vi "Test U8 Change FIFO Size.vi"() -> ()   [LabVIEW 2021]
uses:
  CIFChannels/Typedef/Direction.ctl
  ChannelCommon/typedef/FIFO Config.ctl
  ChannelCommon/typedef/TimeStamps.ctl
  CIF_CIPC_Fifo_U8.lvclass
  D:/dev/Packages/CIF_Channels_Core/src/CIPC_Channels/CIF_CIPC_Chan/CIF_CIPC_Chn.lvclass
  D:/dev/Packages/CIF_Channels_Core/src/CIFChannels/CIFChannels.lvclass
  ChannelCommon/typedef/New FIFO Instance Configuration.ctl
  CIFChannels/CIFChannels.lvclass/CIFChannels.ctl
  CIFChannels/Accessors/Read Publisher Name.vi
  <vilib>/CIF Foundation/CIF Utilities/DataTypes/Flatten Unflatten/Flatten U64.vi
  CIF_CIPC_Chan/CIF_CIPC_Chn.lvclass
  ChannelCommon/ChannelCommon.lvlib
  CIFChannels/CIFChannels.lvclass
panel:
  out "status":string
  out "pass":bool
  out "error out":errorcluster
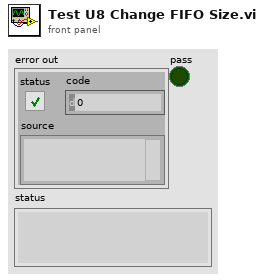
[diagram p1: front panel]
types:
  T1 = typedef "CIFChannels.lvclass/Direction.ctl" = enum16{"Publisher", "Subscriber"}
  T2 = typedef "ChannelCommon.lvlib/New FIFO Instance Configuration.ctl" = cluster{"Backpressure":bool, "Bytes/Message Override":u32, "Messages/FIFO Override":u32, "Custom Data":u8[]}
  T3 = typedef "ChannelCommon.lvlib/TimeStamps.ctl" = cluster{"ClockID":u8, "T0":i64, "T_Out":i64}
  T4 = typedef "ChannelCommon.lvlib/FIFO Config.ctl" = cluster{"Max Bytes/Msg":u64, "Max Msg/FIFO":u64, "Flags":u64}
  T5 = typedef "ChannelCommon.lvlib/New FIFO Instance Response.ctl" = cluster{"Publisher":string, "Custom Data":u8[]}
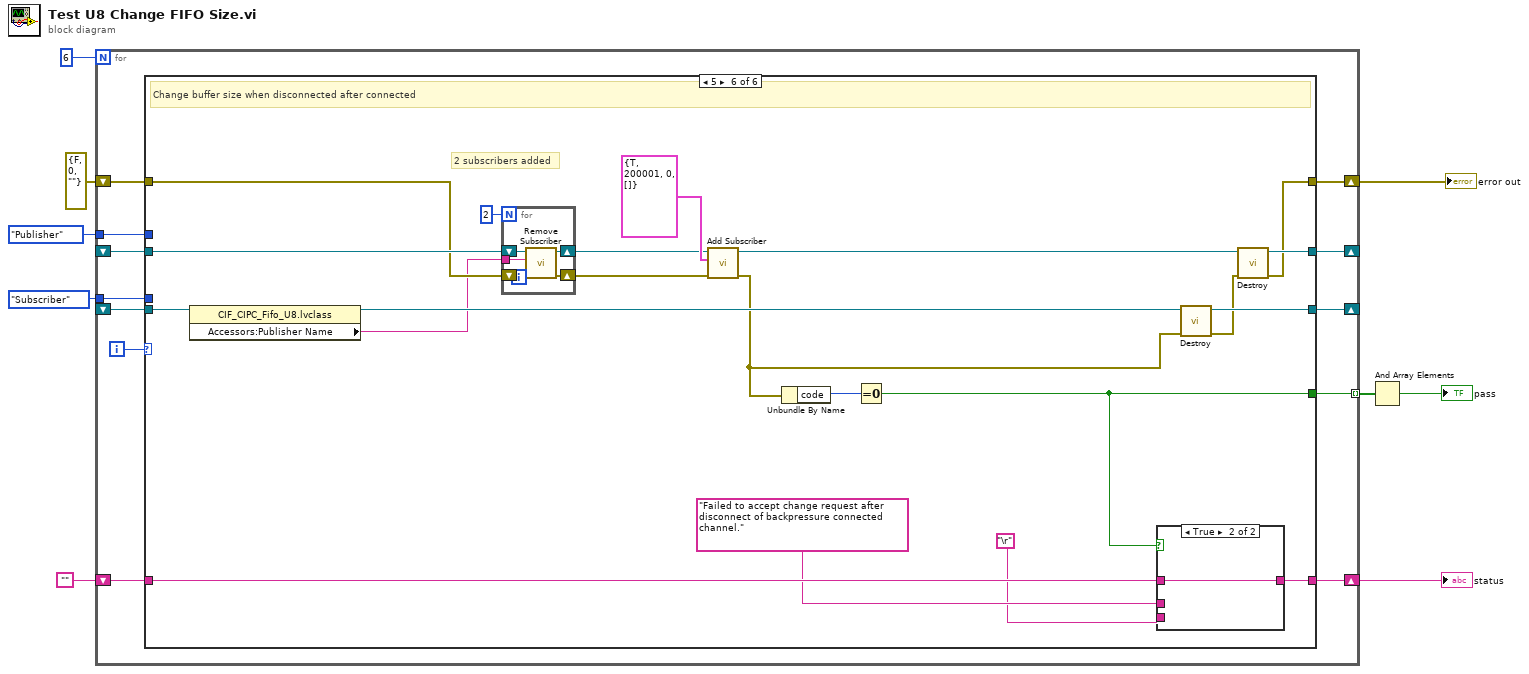
[diagram p0: block diagram]
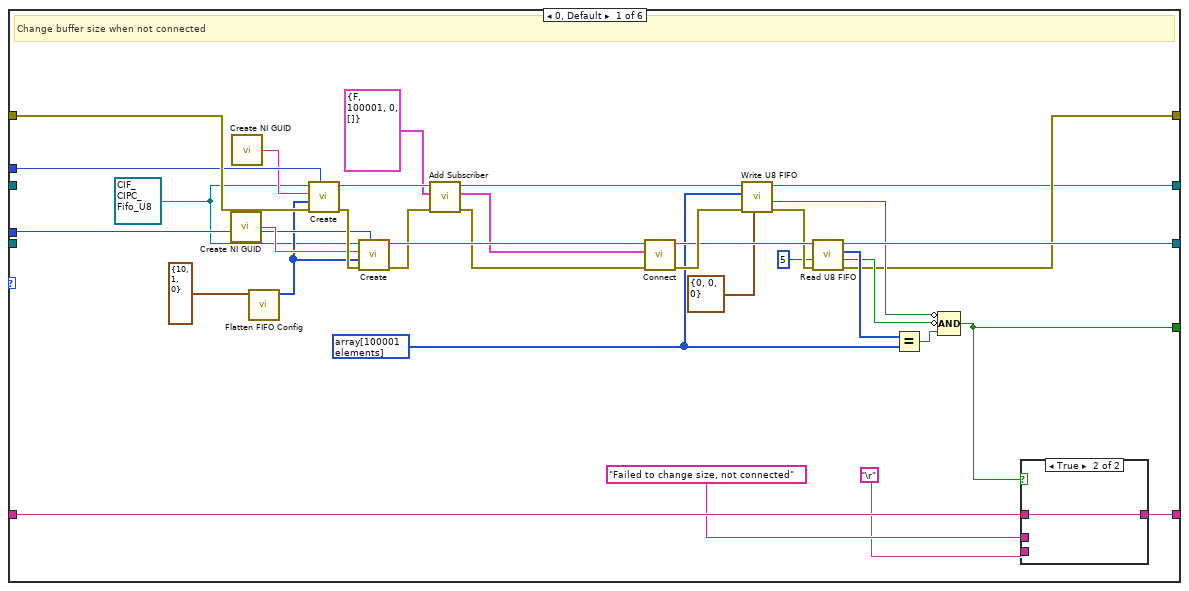
[diagram p2: hidden frame]
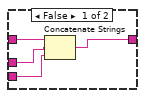
[diagram p3: hidden frame]
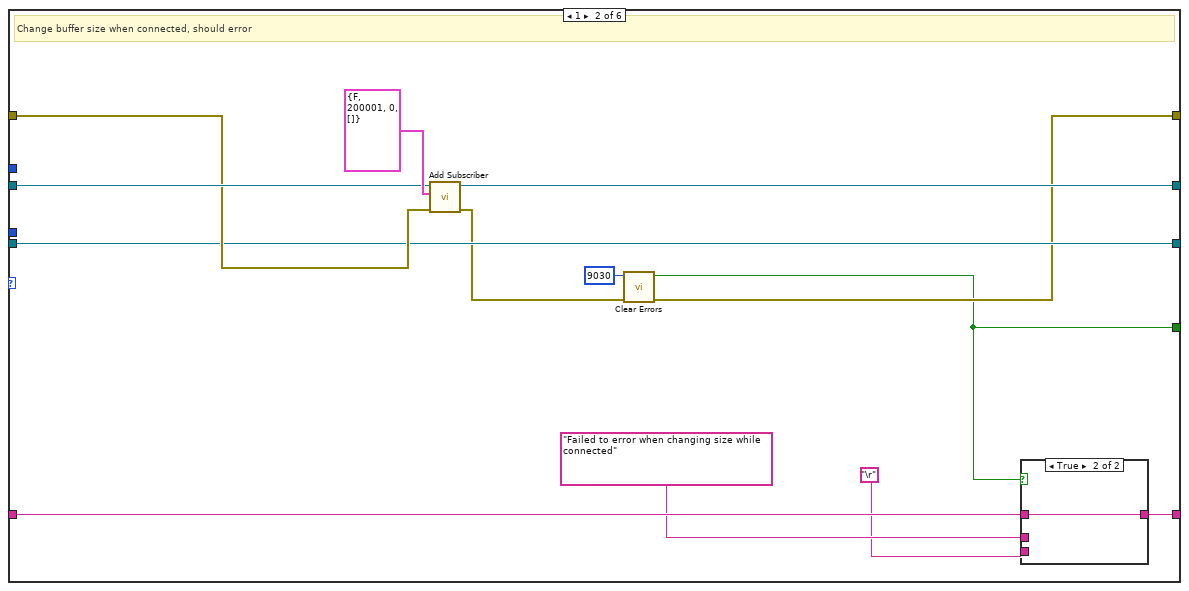
[diagram p4: hidden frame]
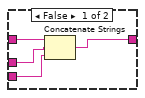
[diagram p5: hidden frame]
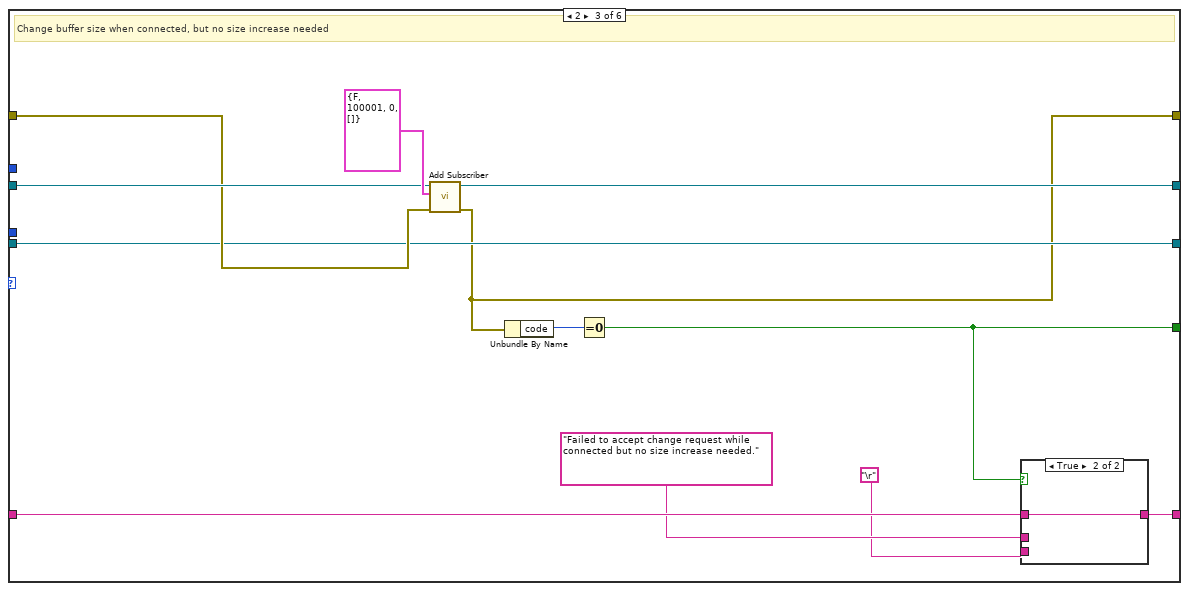
[diagram p6: hidden frame]
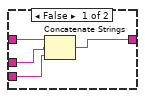
[diagram p7: hidden frame]
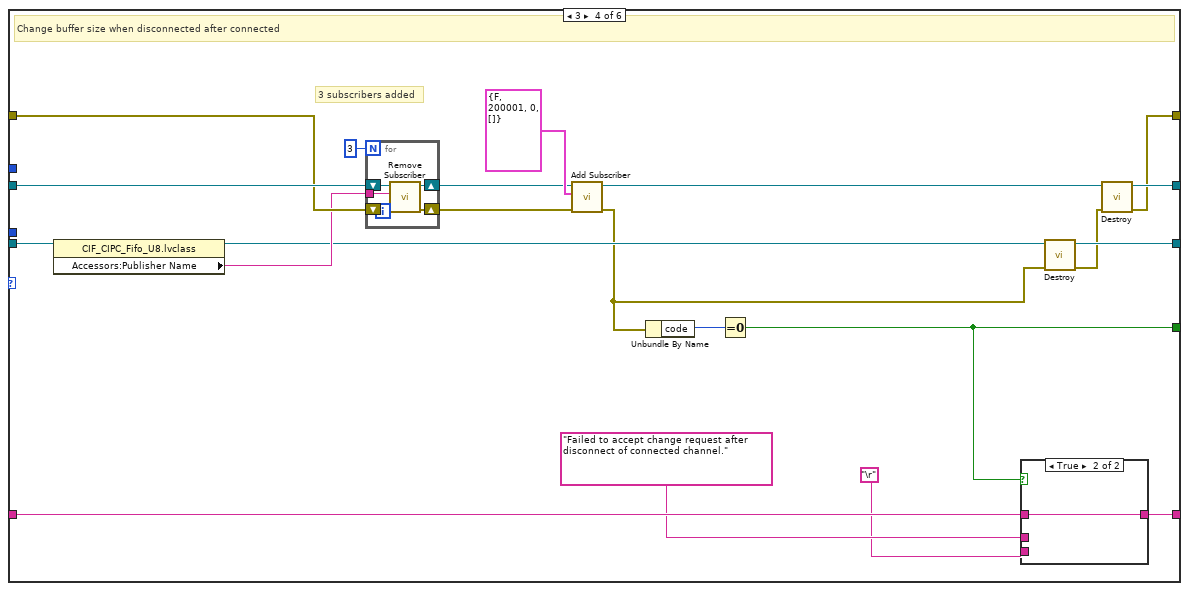
[diagram p8: hidden frame]
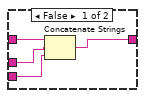
[diagram p9: hidden frame]
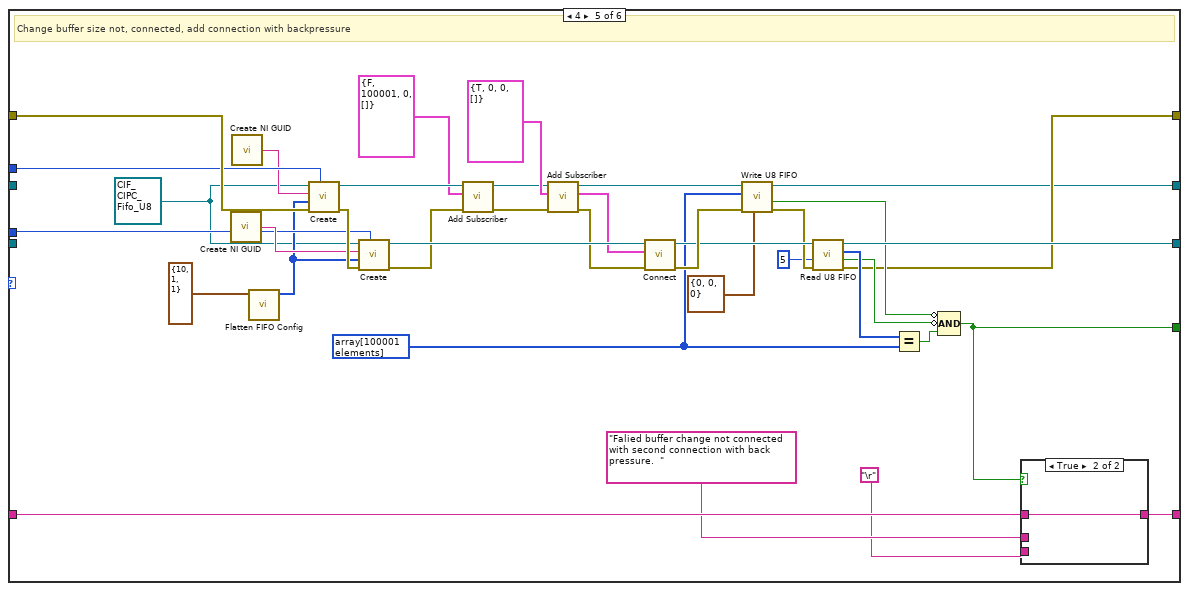
[diagram p10: hidden frame]
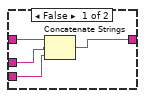
[diagram p11: hidden frame]
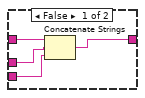
[diagram p12: hidden frame]
diagram:
  n1 = for {
    N: 6 -> [_]
    tunnel: [w21] -> w9 mode=indexing
    shift-right: [w19] -> w1
    shift-left: errorcluster {"status"=FALSE, "code"=0, "source"=""} ("error out") -> [w20]
    shift-right: [w16] -> w5
    shift-left: "" -> [w17]
    tunnel: Direction."Subscriber" ("Direction") -> [w15]
    tunnel: Direction."Publisher" ("Direction") -> [w14]
    shift-right: [w13] -> _
    shift-left: _ -> [w11]
    shift-right: [w12] -> _
    shift-left: _ -> [w10]
    i -> [w18]
    n2 = case shown="5" w18 {
      tunnel: [w50 w61 w79 w110 w158 w183] -> w21
      tunnel: w20 -> [w48 w67 w84 w106 w156 w179]
      tunnel: [w29 w63 w81 w96 w137 w170] -> w19
      tunnel: w17 -> [w55 w73 w90 w116 w163 w189]
      tunnel: [w54 w72 w89 w115 w162 w188] -> w16
      tunnel: w15 -> [w46 _ _ _ w154 _]
      tunnel: w14 -> [w45 _ _ _ w153 _]
      tunnel: [w39 w66 w83 w100 w147 w174] -> w13
      tunnel: [w28 w65 w82 w99 w136 w173] -> w12
      tunnel: w10 -> [_ w68 w85 w109 _ w182]
      tunnel: w11 -> [_ w66 w83 w105 _ w178]
      frame 0, Default {
        w33 = refnum<class "CIF_CIPC_Fifo_U8.lvclass"> refnum ("CIF_CIPC_Fifo_U8.lvclass")
        w30 = u8[] array[100001 elements] ("U8 Data")
        # "Change buffer size when not connected"
        n3 = call <vilib>:"Create NI GUID.vi"() -> ("NI GUID"=w47:string)
        n4 = call <vilib>:"Create NI GUID.vi"() -> ("NI GUID"=w43:string)
        n5 = call "Flatten FIFO Config.vi"("FIFO Config in"=T4 {"Max Bytes/Msg"=10, "Max Msg/FIFO"=1, "Flags"=0}) -> ("Flattened FIFO Config"=w34:u8[])  [unwired: 10 in]
        n6 = call-dynamic "Create.vi"("Direction"=w45, "error in (no error)"=w48, "Custom Config Data"=w34, "Name"=w43, "CIFFIFO in"=w33) -> ("error out"=w49:errorcluster, "CIFFIFO out"=w27:refnum<class "CIF_CIPC_Fifo_U8.lvclass">)  [unwired: 5 in]
        n7 = call-dynamic "Create.vi"("Direction"=w46, "error in (no error)"=w49, "Custom Config Data"=w34, "Name"=w47, "CIFFIFO in"=w33) -> ("error out"=w23:errorcluster, "CIFFIFO out"=w42:refnum<class "CIF_CIPC_Fifo_U8.lvclass">)  [unwired: 5 in]
        n8 = call-dynamic "Add Subscriber.vi"("error in (no error)"=w23, "New FIFO Instance Config"=T2 {"Backpressure"=FALSE, "Bytes/Message Override"=100001, "Messages/FIFO Override"=0, "Custom Data"=[]}, "CIF_CIPC_Chn in"=w27) -> ("error out"=w22:errorcluster, "New FIFO Instance"=w25:T5, "CIF_CIPC_Chn out"=w26:refnum<class "CIF_CIPC_Fifo_U8.lvclass">)  [unwired: 6 in]
        n9 = call-dynamic "Connect.vi"("error in (no error)"=w22, "Connection"=w25, "CIFTag in"=w42) -> ("error out"=w41:errorcluster, "CIFTag out"=w40:refnum<class "CIF_CIPC_Fifo_U8.lvclass">)  [unwired: 7 in]
        n10 = call-dynamic "Write U8 FIFO.vi"("FIFO Timestamps"=T3 {"ClockID"=0, "T0"=0, "T_Out"=0}, "error in (no error)"=w41, "Data in"=w30, "CIFFIFO in"=w26) -> ("error out"=w38:errorcluster, "timed out?"=w37:bool, "CIFFIFO out"=w28:refnum<class "CIF_CIPC_Fifo_U8.lvclass">)  [unwired: 4 in, 1 out]
        n11 = call-dynamic "Read U8 FIFO.vi"("error in (no error)"=w38, "Timeout (ms)"=5, "CIFFIFO in"=w40) -> ("error out"=w29:errorcluster, "timed out?"=w35:bool, "Data out"=w36:u8[], "CIFFIFO out"=w39:refnum<class "CIF_CIPC_Fifo_U8.lvclass">)  [unwired: 4 in, 1 out]
        n12 = Equal?(x=w36, y=w30) -> (x = y?=w51:bool)
        n13 = Compound Arithmetic op=AND(invert w37, invert w35, w51) -> (w50:bool)
        n14 = case shown="True" w50 {
          tunnel: w55 -> [w59 w60]
          tunnel: [w56 w60] -> w54
          tunnel: "Failed to change size, not connected" -> [w58 _]
          tunnel: "\r" -> [w57 _]
          frame False {
            n15 = Concatenate Strings(w59, w58, w57) -> (w56:string)
          }
          frame True {
          }
        }
      }
      frame 1 {
        # "Change buffer size when connected, should error"
        n16 = call-dynamic "Add Subscriber.vi"("error in (no error)"=w67, "New FIFO Instance Config"=T2 {"Backpressure"=FALSE, "Bytes/Message Override"=200001, "Messages/FIFO Override"=0, "Custom Data"=[]}, "CIF_CIPC_Chn in"=w68) -> ("error out"=w64:errorcluster, "CIF_CIPC_Chn out"=w65:refnum<class "CIF_CIPC_Chn.lvclass">)  [unwired: 6 in, 1 out]
        n17 = call <vilib>:"Clear Errors.vi"("error in (no error)"=w64, "specific error code to clear (0: all)"=9030) -> ("error out"=w63:errorcluster, "specific error cleared?"=w61:bool)  [unwired: 4 in]
        n18 = case shown="True" w61 {
          tunnel: w73 -> [w77 w78]
          tunnel: [w74 w78] -> w72
          tunnel: "Failed to error when changing size while connected" -> [w76 _]
          tunnel: "\r" -> [w75 _]
          frame False {
            n19 = Concatenate Strings(w77, w76, w75) -> (w74:string)
          }
          frame True {
          }
        }
      }
      frame 2 {
        # "Change buffer size when connected, but no size increase needed"
        n20 = call-dynamic "Add Subscriber.vi"("error in (no error)"=w84, "New FIFO Instance Config"=T2 {"Backpressure"=FALSE, "Bytes/Message Override"=100001, "Messages/FIFO Override"=0, "Custom Data"=[]}, "CIF_CIPC_Chn in"=w85) -> ("error out"=w81:errorcluster, "CIF_CIPC_Chn out"=w82:refnum<class "CIF_CIPC_Chn.lvclass">)  [unwired: 6 in, 1 out]
        n21 = Unbundle By Name(w81) -> ("code"=w80:i32)
        n22 = Equal To 0?(x=w80) -> (x = 0?=w79:bool)
        n23 = case shown="True" w79 {
          tunnel: w90 -> [w94 w95]
          tunnel: [w91 w95] -> w89
          tunnel: "Failed to accept change request while connected but no size increase needed." -> [w93 _]
          tunnel: "\r" -> [w92 _]
          frame False {
            n24 = Concatenate Strings(w94, w93, w92) -> (w91:string)
          }
          frame True {
          }
        }
      }
      frame 3 {
        # "3 subscribers added"
        # "Change buffer size when disconnected after connected"
        n25 = property class="CIF_CIPC_Fifo_U8.lvclass"(reference=w105) -> (reference out=w101:refnum<class "CIF_CIPC_Fifo_U8.lvclass">, "Accessors:Publisher Name"=w104:string)  [unwired: 1 in, 1 out]
        n26 = for {
          N: 3 -> [_]
          tunnel: w104 -> [w117]
          shift-right: [w119] -> w107
          shift-left: w106 -> [w118]
          shift-right: [w120] -> w108
          shift-left: w109 -> [w121]
          n27 = call-dynamic "Remove Subscriber.vi"("error in (no error)"=w118, "Publisher to Remove"=w117, "CIF_CIPC_Chn in"=w121) -> ("error out"=w119:errorcluster, "CIF_CIPC_Chn out"=w120:refnum<class "CIF_CIPC_Chn.lvclass">)  [unwired: 7 in]
        }
        n28 = call-dynamic "Add Subscriber.vi"("error in (no error)"=w107, "New FIFO Instance Config"=T2 {"Backpressure"=FALSE, "Bytes/Message Override"=200001, "Messages/FIFO Override"=0, "Custom Data"=[]}, "CIF_CIPC_Chn in"=w108) -> ("error out"=w98:errorcluster, "CIF_CIPC_Chn out"=w102:refnum<class "CIF_CIPC_Chn.lvclass">)  [unwired: 6 in, 1 out]
        n29 = Unbundle By Name(w98) -> ("code"=w111:i32)
        n30 = Equal To 0?(x=w111) -> (x = 0?=w110:bool)
        n31 = case shown="True" w110 {
          tunnel: w116 -> [w125 w126]
          tunnel: [w122 w126] -> w115
          tunnel: "Failed to accept change request after disconnect of connected channel." -> [w124 _]
          tunnel: "\r" -> [w123 _]
          frame False {
            n32 = Concatenate Strings(w125, w124, w123) -> (w122:string)
          }
          frame True {
          }
        }
        n33 = call-dynamic "Destroy.vi"("error in (no error)"=w98, "CIFTag in"=w101) -> ("error out"=w97:errorcluster, "CIFTag out"=w100:refnum<class "CIF_CIPC_Fifo_U8.lvclass">)  [unwired: 8 in]
        n34 = call-dynamic "Destroy.vi"("error in (no error)"=w97, "CIFTag in"=w102) -> ("error out"=w96:errorcluster, "CIFTag out"=w99:refnum<class "CIF_CIPC_Chn.lvclass">)  [unwired: 8 in]
      }
      frame 4 {
        w141 = refnum<class "CIF_CIPC_Fifo_U8.lvclass"> refnum ("CIF_CIPC_Fifo_U8.lvclass")
        w138 = u8[] array[100001 elements] ("U8 Data")
        # "Change buffer size not, connected, add connection with backpressure"
        n35 = call <vilib>:"Create NI GUID.vi"() -> ("NI GUID"=w155:string)
        n36 = call <vilib>:"Create NI GUID.vi"() -> ("NI GUID"=w151:string)
        n37 = call "Flatten FIFO Config.vi"("FIFO Config in"=T4 {"Max Bytes/Msg"=10, "Max Msg/FIFO"=1, "Flags"=1}) -> ("Flattened FIFO Config"=w142:u8[])  [unwired: 10 in]
        n38 = call-dynamic "Create.vi"("Direction"=w153, "error in (no error)"=w156, "Custom Config Data"=w142, "Name"=w151, "CIFFIFO in"=w141) -> ("error out"=w157:errorcluster, "CIFFIFO out"=w131:refnum<class "CIF_CIPC_Fifo_U8.lvclass">)  [unwired: 5 in]
        n39 = call-dynamic "Create.vi"("Direction"=w154, "error in (no error)"=w157, "Custom Config Data"=w142, "Name"=w155, "CIFFIFO in"=w141) -> ("error out"=w128:errorcluster, "CIFFIFO out"=w150:refnum<class "CIF_CIPC_Fifo_U8.lvclass">)  [unwired: 5 in]
        n40 = call-dynamic "Add Subscriber.vi"("error in (no error)"=w128, "New FIFO Instance Config"=T2 {"Backpressure"=FALSE, "Bytes/Message Override"=100001, "Messages/FIFO Override"=0, "Custom Data"=[]}, "CIF_CIPC_Chn in"=w131) -> ("error out"=w129:errorcluster, "CIF_CIPC_Chn out"=w130:refnum<class "CIF_CIPC_Fifo_U8.lvclass">)  [unwired: 6 in, 1 out]
        n41 = call-dynamic "Add Subscriber.vi"("error in (no error)"=w129, "New FIFO Instance Config"=T2 {"Backpressure"=TRUE, "Bytes/Message Override"=0, "Messages/FIFO Override"=0, "Custom Data"=[]}, "CIF_CIPC_Chn in"=w130) -> ("error out"=w132:errorcluster, "New FIFO Instance"=w134:T5, "CIF_CIPC_Chn out"=w135:refnum<class "CIF_CIPC_Fifo_U8.lvclass">)  [unwired: 6 in]
        n42 = call-dynamic "Connect.vi"("error in (no error)"=w132, "Connection"=w134, "CIFTag in"=w150) -> ("error out"=w149:errorcluster, "CIFTag out"=w148:refnum<class "CIF_CIPC_Fifo_U8.lvclass">)  [unwired: 7 in]
        n43 = call-dynamic "Write U8 FIFO.vi"("FIFO Timestamps"=T3 {"ClockID"=0, "T0"=0, "T_Out"=0}, "error in (no error)"=w149, "Data in"=w138, "CIFFIFO in"=w135) -> ("error out"=w146:errorcluster, "timed out?"=w145:bool, "CIFFIFO out"=w136:refnum<class "CIF_CIPC_Fifo_U8.lvclass">)  [unwired: 4 in, 1 out]
        n44 = call-dynamic "Read U8 FIFO.vi"("error in (no error)"=w146, "Timeout (ms)"=5, "CIFFIFO in"=w148) -> ("error out"=w137:errorcluster, "timed out?"=w143:bool, "Data out"=w144:u8[], "CIFFIFO out"=w147:refnum<class "CIF_CIPC_Fifo_U8.lvclass">)  [unwired: 4 in, 1 out]
        n45 = Equal?(x=w144, y=w138) -> (x = y?=w159:bool)
        n46 = Compound Arithmetic op=AND(invert w145, invert w143, w159) -> (w158:bool)
        n47 = case shown="True" w158 {
          tunnel: w163 -> [w167 w168]
          tunnel: [w164 w168] -> w162
          tunnel: "Falied buffer change not connected with second connection with back pressure.  " -> [w166 _]
          tunnel: "\r" -> [w165 _]
          frame False {
            n48 = Concatenate Strings(w167, w166, w165) -> (w164:string)
          }
          frame True {
          }
        }
      }
      frame 5 {
        # "2 subscribers added"
        # "Change buffer size when disconnected after connected"
        n49 = property class="CIF_CIPC_Fifo_U8.lvclass"(reference=w178) -> (reference out=w175:refnum<class "CIF_CIPC_Fifo_U8.lvclass">, "Accessors:Publisher Name"=w169:string)  [unwired: 1 in, 1 out]
        n50 = for {
          N: 2 -> [_]
          tunnel: w169 -> [w190]
          shift-right: [w192] -> w180
          shift-left: w179 -> [w191]
          shift-right: [w193] -> w181
          shift-left: w182 -> [w194]
          n51 = call-dynamic "Remove Subscriber.vi"("error in (no error)"=w191, "Publisher to Remove"=w190, "CIF_CIPC_Chn in"=w194) -> ("error out"=w192:errorcluster, "CIF_CIPC_Chn out"=w193:refnum<class "CIF_CIPC_Chn.lvclass">)  [unwired: 7 in]
        }
        n52 = call-dynamic "Add Subscriber.vi"("error in (no error)"=w180, "New FIFO Instance Config"=T2 {"Backpressure"=TRUE, "Bytes/Message Override"=200001, "Messages/FIFO Override"=0, "Custom Data"=[]}, "CIF_CIPC_Chn in"=w181) -> ("error out"=w172:errorcluster, "CIF_CIPC_Chn out"=w176:refnum<class "CIF_CIPC_Chn.lvclass">)  [unwired: 6 in, 1 out]
        n53 = Unbundle By Name(w172) -> ("code"=w184:i32)
        n54 = Equal To 0?(x=w184) -> (x = 0?=w183:bool)
        n55 = case shown="True" w183 {
          tunnel: w189 -> [w198 w199]
          tunnel: [w195 w199] -> w188
          tunnel: "Failed to accept change request after disconnect of backpressure connected channel." -> [w197 _]
          tunnel: "\r" -> [w196 _]
          frame False {
            n56 = Concatenate Strings(w198, w197, w196) -> (w195:string)
          }
          frame True {
          }
        }
        n57 = call-dynamic "Destroy.vi"("error in (no error)"=w172, "CIFTag in"=w175) -> ("error out"=w171:errorcluster, "CIFTag out"=w174:refnum<class "CIF_CIPC_Fifo_U8.lvclass">)  [unwired: 8 in]
        n58 = call-dynamic "Destroy.vi"("error in (no error)"=w171, "CIFTag in"=w176) -> ("error out"=w170:errorcluster, "CIFTag out"=w173:refnum<class "CIF_CIPC_Chn.lvclass">)  [unwired: 8 in]
      }
    }
  }
  "error out" <- w1
  "status" <- w5
  n59 = And Array Elements(Boolean array=w9) -> (logical AND=→"pass":bool)
